vi "Pcre2SetDepthLimit8.vi"(8 "error in":errorcluster, 10 "DepthLimit":u32, 11 "pMatchContext":u64 format="%.0x") -> (0 "error out":errorcluster, 3 "pMatchContext":u64 format="%.0x")   [LabVIEW 2021, in "libpcre2-8.lvlib"]
uses:
  libpcre2-8.lvlib
  libpcre2-8-x32.dll
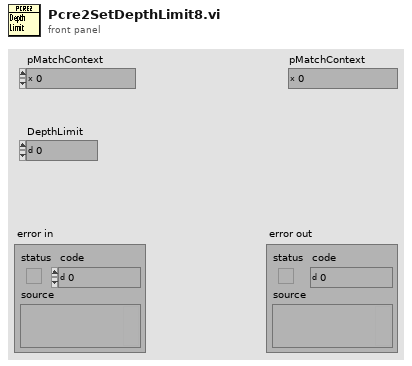
[diagram p1: front panel]
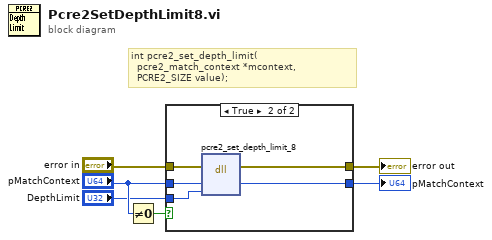
[diagram p0: block diagram]
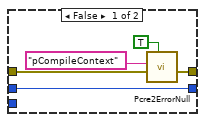
[diagram p2: hidden frame]
diagram:
  # "int pcre2_set_depth_limit(\n  pcre2_match_context *mcontext,\n  PCRE2_SIZE value);"
  n1 = Not Equal To 0?(x="pMatchContext") -> (x != 0?=w1:bool)
  n2 = case shown="True" w1 {
    tunnel: "error in" -> [w10 w16]
    tunnel: [w11 w15] -> w5
    tunnel: "DepthLimit" -> [_ w14]
    tunnel: "pMatchContext" -> [w8 w13]
    tunnel: [w8 w12] -> w4
    frame False {
      n3 = call "Pcre2ErrorNull.vi"("IsPointer? (F)"=TRUE, "error in"=w10, "What"="pCompileContext") -> ("error out"=w11:errorcluster)  [unwired: 8 in]
    }
    frame True {
      n4 = dll-call lib="libpcre2-8-x*.dll" fn="pcre2_set_depth_limit_8"(error in=w16, "mcontext"=w13, "value"=w14) -> (error out=w15:errorcluster, "mcontext"=w12:u64)  [unwired: 4 in, 1 out]
    }
  }
  "error out" <- w5
  "pMatchContext" <- w4
